vi "Get DAQ DI ScanArray Data.vi"(0 "DAQ":refnum<class "DAQ.lvclass">, 11 "error in (no error)":errorcluster) -> (4 "DAQ":refnum<class "DAQ.lvclass">, 6 "DI ScanArray":bool[](array[boolean]), 8 "Timestamp (DBL)":dbl, 10 "Time Stamp":timestamp, 15 "error out":errorcluster)   [LabVIEW 2022 SP3, in "DAQ.lvclass"]
doc: "Developed by Kevin Thompson\nkevin@thompsonengineering.net\n\nCopyright 2018-2020\nThompson Engineering, LLC\nThis public method retrieves the scanned digital inputs (DI) as an array, in the order of the DI IOName TD enum."
uses:
  DAQ.lvclass
  Process/ProcessSupport/TD DaqThread--enum.ctl
  DAQ.lvclass/DAQ.ctl
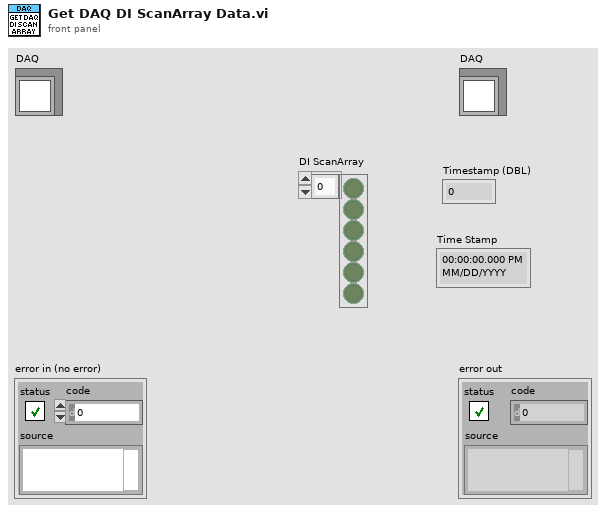
[diagram p1: front panel]
types:
  T1 = typedef "DAQ.lvclass/TD DaqThread--enum.ctl" = enum16{"AI", "DI"}
  T2 = typedef "TD Dynamic CVT DVR--ref.ctl" = refnum<data-value>
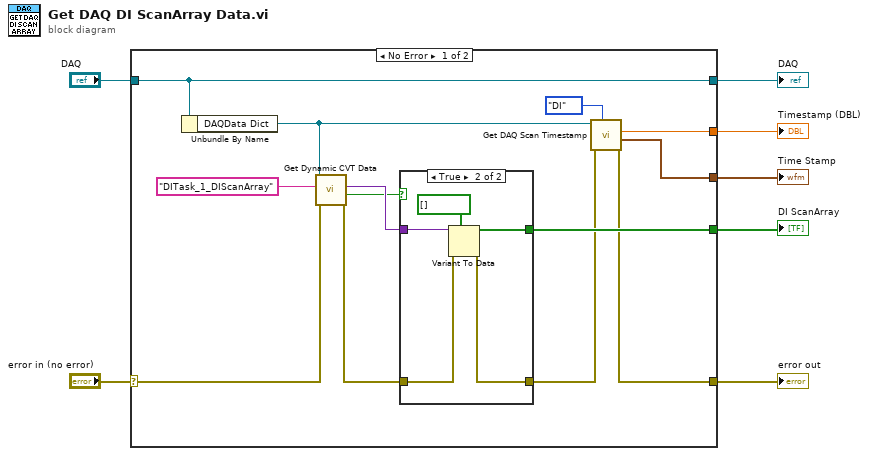
[diagram p0: block diagram]
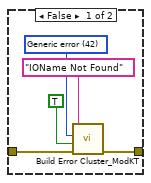
[diagram p2: hidden frame]
diagram:
  n1 = case shown="No Error" "error in (no error)" {
    selector: "error in (no error)" -> [w14 w32]
    tunnel: [w11 w32] -> w6
    tunnel: [w20 w31] -> w4
    tunnel: "DAQ" -> [w20 w31]
    tunnel: [w16 _] -> w3
    tunnel: [w9 _] -> w2
    tunnel: [w8 _] -> w1
    frame No Error {
      n2 = Unbundle By Name(w20) -> ("DAQData Dict"=w12:T2)
      n3 = call <vilib>:"Get Dynamic CVT Data.vi"("error in (no error)"=w14, "DataName"="DITask_1_DIScanArray", "dCVT DVR"=w12) -> ("error out"=w19:errorcluster, "found"=w17:bool, "value"=w18:variant)  [unwired: 5 in, 1 out]
      n4 = case shown="True" w17 {
        tunnel: w19 -> [w22 w30]
        tunnel: [w21 w29] -> w10
        tunnel: w18 -> [_ w28]
        tunnel: [_ w27] -> w16
        frame False {
          w24 = 42 items=["No error", "Argument error", "Memory is full", "Out of zone", "End of file", "File already open", "Generic file I/O error", "File not found", "File permission error", "Disk is full", "Duplicate path", "Too many files open", "System feature not enabled", "Resource file not found", "Cannot add resource", "Resource not found", "Image not found", "Image memory error", "Pen does not exist", "Config type invalid", "Config token not found", "Config parse error", "Config memory error", "Bad external code format", "Bad external code offset", "External code not present", "Null window", "Destroy window error", "Null menu", "Print aborted", "Bad print record", "Print driver error", "Windows error during printing", "Memory error during printing", "Print dialog error", "Generic print error", "Invalid device refnum", "Device not found", "Device parameter error", "Device unit error", "Cannot open device", "Device call aborted", "Generic error", "Cancelled by user", "Object ID too low", "Object ID too high", "Object not in heap", "Unknown heap", "Unknown object (invalid DefProc)", "Unknown object (DefProc not in table)", "Message out of range", "Invalid (null) method", "Unknown message", "Manager call not supported", "Bad address", "Network operation in progress", "Network operation timed out", "Connection is busy", "Network attribute not supported", "Network error", "Address in use", "System out of memory", "Connection aborted", "Connection refused", "Not connected", "Already connected", "Connection closed", "Initialization error (interapplication manager)", "Bad occurrence", "Wait on unbound occurrence handler", "Occurrence queue overflow", "Datalog type conflict", "Unused", "Unrecognized type (interapplication manager)", "Memory corrupt", "Failed to make temporary DLL", "Old CIN version", "Drag socket not found", "Failed to load drop-object", "Failed to register OLE object", "Failed to release OLE object", "Format specifier type mismatch", "Unknown format specifier", "Too few format specifiers", "Too many format specifiers", "Scan failed", "Newer CIN version", "Error converting to variant", "Runtime menu error", "Password tampered", "Variant attribute not found", "Incompatible variant data type", "Event data is not available", "Event Store is not present", "Occurrence is not found", "Event Queue is not created", "Event info is not available", "Refnum passed is NULL", "Error retrieving Class GUID", "Error retrieving CoClass GUID", "Error retrieving TypeLib GUID.", "Bad built application magic bytes.", "Specific driver is different from the specific driver associated with the Logical Name.", "There is no session opened to the class driver.", "Max Error", "MAX - Error with config objects", "MAX - Error loading configuration", "MAX - Group not supported"]
          n5 = call <vilib>:"Build Error Cluster_ModKT .vi"("Prepend String (\"\")"="IOName Not Found" ("Prepend String (\"\")"), "code"=w24, "error? (F)"=TRUE, "error in (no error)"=w22) -> ("error out"=w21:errorcluster)  [unwired: 3 in, 1 out]
        }
        frame True {
          n6 = Variant To Data(error in=w30, type=bool[] [], Variant=w28) -> (data=w27:bool[], error out=w29:errorcluster)
        }
      }
      n7 = call "Get DAQ Scan Timestamp.vi"("Daq Thread"=TD_DaqThread--enum."DI", "error in (no error)"=w10, "DaqData dCVT"=w12) -> ("error out"=w11:errorcluster, "Time Stamp"=w8:timestamp, "Timestamp (DBL)"=w9:dbl)  [unwired: 5 in, 1 out]
    }
    frame Error {
    }
  }
  "error out" <- w6
  "DAQ" <- w4
  "DI ScanArray" <- w3
  "Time Stamp" <- w1
  "Timestamp (DBL)" <- w2
